vi "Accumulate Array.vi"(6 "initial":dbl[](array[numeric]), 8 "Reset?":bool, 9 "value":dbl) -> (1 "output array":dbl[](array[numeric]))   [LabVIEW 2020]
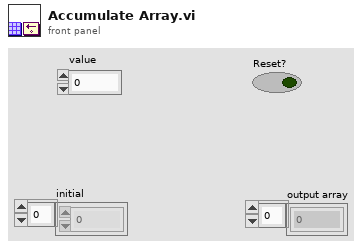
[diagram p1: front panel]
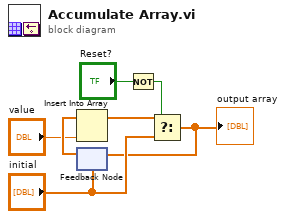
[diagram p0: block diagram]
diagram:
  n1 = feedback #1("initial") -> (w7:dbl[])
  n2 = Insert Into Array(array=w7, new element="value") -> (w4:dbl[])  [unwired: 1 in]
  n3 = Not(x="Reset?") -> (.not. x?=w3:bool)
  n4 = Select(t=w4, s=w3, f="initial") -> (s? t:f=w1:dbl[])
  "output array" <- w1
  n5 = feedback-in #1(w1) -> ()
